vi "Write Channel Ref.vi"(8 "error in (no error)":errorcluster, 10 "Device Item Ref":T1=18446744073709551615 format="%.0x", 11 "Configuration.Channel in":refnum<class "Configuration.Channel.lvclass">) -> (0 "error out":errorcluster, 3 "Configuration.Channel out":refnum<class "Configuration.Channel.lvclass">)   [LabVIEW 2016, in "Configuration.Channel.lvclass"]
uses:
  Configuration.Channel.lvclass
  <vilib>/NI Veristand/Custom Device API/Custom Device Item Ref.ctl
  Configuration.Channel.lvclass/Configuration.Channel.ctl
  <vilib>/NI VeriStand/Custom Device API/Custom Device API.lvlib
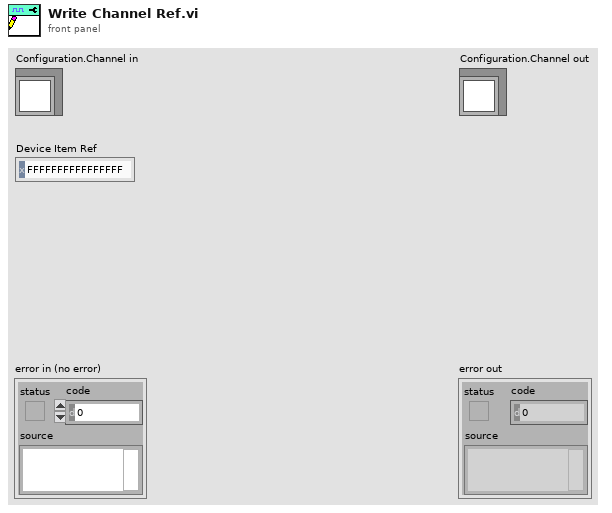
[diagram p1: front panel]
types:
  T1 = typedef "Custom Device API.lvlib/Custom Device Item Ref.ctl" = u64
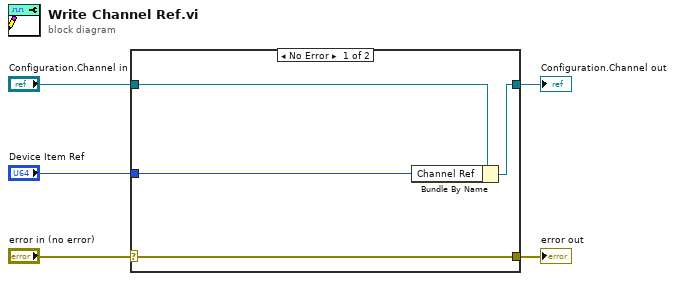
[diagram p0: block diagram]
diagram:
  n1 = case shown="No Error" "error in (no error)" {
    selector: "error in (no error)" -> [w9 w10]
    tunnel: [w9 w10] -> w4
    tunnel: [w7 w11] -> w2
    tunnel: "Configuration.Channel in" -> [w8 w11]
    tunnel: "Device Item Ref" -> [w6 _]
    frame No Error {
      n2 = Bundle By Name(cluster=w8, "Channel Ref"=w6) -> (w7:refnum<class "Configuration.Channel.lvclass">)
    }
    frame Error {
    }
  }
  "error out" <- w4
  "Configuration.Channel out" <- w2
